vi "Write JSON Config.vi"(6 "Pretty Print?":bool, 8 "error in (no error)":errorcluster, 11 "AbsComp_One Term_CPLX_EXT in":refnum<class "AbsComp_One Term_CPLX_EXT.lvclass">) -> (0 "error out":errorcluster, 2 "JSON":string, 3 "AbsComp_One Term_CPLX_EXT out":refnum<class "AbsComp_One Term_CPLX_EXT.lvclass">)   [LabVIEW 2021, in "AbsComp_One Term_CPLX_EXT.lvclass"]
uses:
  AbsComp_One Term_CPLX_EXT.lvclass
  C:/Program Files (x86)/National Instruments/LabVIEW 2021/vi.lib/TSA/Abstract Data Classes/Abs_Types/Type/Abs_Type.lvclass
  AbsComp_One Term_CPLX_EXT.lvclass/AbsComp_One Term_CPLX_EXT.ctl
  <vilib>/JDP Science/JSONtext/Make JSON Array.vi
  <vilib>/JDP Science/JSONtext/Merge into Object.vi
  <vilib>/JDP Science/JSONtext/Make JSON Object.vi
  <vilib>/Utility/LVClass/Get LV Class Name.vi
  <vilib>/JDP Science/JSONtext/support/Format JSON Array Text.vi
  <vilib>/JDP Science/JSONtext/support/Format JSON Object.vi
  <vilib>/JDP Science/JSONtext/Get all Object Items.vi
  <vilib>/JDP Science/JSONtext/Set Multiple Object Items.vi
  Abs_Types/Complex Extended Float/Abs_Complex Extended Float.lvclass
  Abs_Types/Boolean/Abs_Boolean.lvclass
  Abs_Types/Type/Abs_Type.lvclass
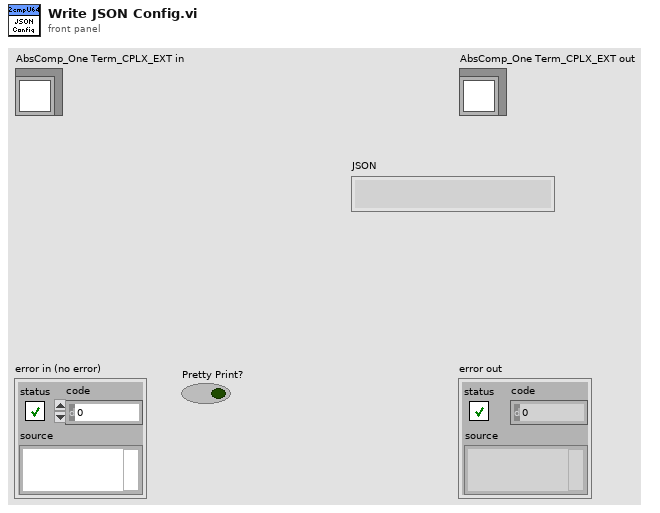
[diagram p1: front panel]
types:
  T1 = typedef "AbsComp_One Term_CPLX_EXT.lvclass/Abstract Type.ctl" = refnum<class "Abs_Complex Extended Float.lvclass">
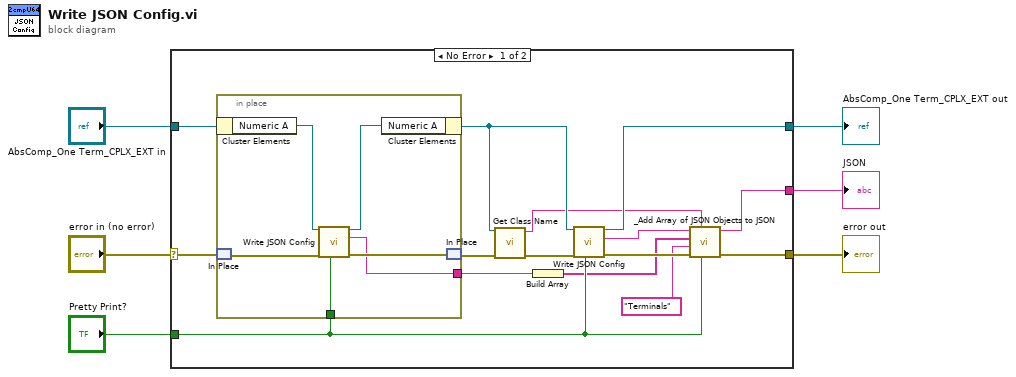
[diagram p0: block diagram]
diagram:
  n1 = case shown="No Error" "error in (no error)" {
    selector: "error in (no error)" -> [w17 w29]
    tunnel: "AbsComp_One Term_CPLX_EXT in" -> [w21 w28]
    tunnel: [w20 w28] -> w3
    tunnel: [w13 _] -> w4
    tunnel: [w12 w29] -> w5
    tunnel: "Pretty Print?" -> [w11 _]
    frame No Error {
      n2 = in-place {
        in-place-border: w11 -> [w26]
        in-place-border: [w24] -> w19
        n3 = in-place-cluster #1(w21) -> ("Numeric A"=w23:T1)
        n4 = in-place-match #2(w17) -> (w27:errorcluster)
        n5 = call-dynamic "Write JSON Config.vi"("Pretty Print?"=w26, "error in (no error)"=w27, "Abs_Type in"=w23) -> ("error out"=w25:errorcluster, "JSON"=w24:string, "Abs_Type out"=w22:T1)  [unwired: 6 in]
        n6 = in-place-cluster #1("Numeric A"=w22) -> (w15:refnum<class "AbsComp_One Term_CPLX_EXT.lvclass">)
        n7 = in-place-match #2(w25) -> (w18:errorcluster)
      }
      n8 = call "Get Class Name.vi"("error in (no error)"=w18, "Abs_Type in"=w15) -> ("error out"=w16:errorcluster, "class name"=w10:string)  [unwired: 8 in]
      n9 = Build Array(w19) -> (w8:string[])
      n10 = call-parent "Write JSON Config.vi"("Pretty Print?"=w11, "error in (no error)"=w16, "Abs_Type in"=w15) -> ("error out"=w14:errorcluster, "JSON"=w9:string, "Abs_Type out"=w20:refnum<class "AbsComp_One Term_CPLX_EXT.lvclass">)  [unwired: 6 in]
      n11 = call "_Add Array of JSON Objects to JSON.vi"("Pretty Print?"=w11, "JSON Object Name"=w10, "error in (no error)"=w14, "JSON Array Name"="Terminals", "JSON Objects"=w8, "JSON"=w9) -> ("error out"=w12:errorcluster, "<JSON>"=w13:string)  [unwired: 4 in]
    }
    frame Error {
    }
  }
  "error out" <- w5
  "AbsComp_One Term_CPLX_EXT out" <- w3
  "JSON" <- w4
